vi "Create simplified GUI element.vi"(8 "error in (no error)":errorcluster, 10 "Index":i32, 11 "Optimiser SBlock in":refnum<class "Optimiser SBlock.lvclass">) -> (0 "error out":errorcluster, 2 "Simple GUI Element":T1={"Bcg Color"=16777225, "Index"=0, "No. of runs"=0, "Script name"="", "FPGA name"="", "Parameters"="", "Repetitions"=0}, 3 "Optimiser SBlock out":refnum<class "Optimiser SBlock.lvclass">)   [LabVIEW 2020, in "Run Utilities.lvlib" / "Optimiser SBlock.lvclass"]
doc: "Create a GUI element for this SBlock"
uses:
  Optimiser SBlock.lvclass
  Schedule Block/Schedule Block.lvclass
  Optimiser SBlock.lvclass/Optimiser SBlock.ctl
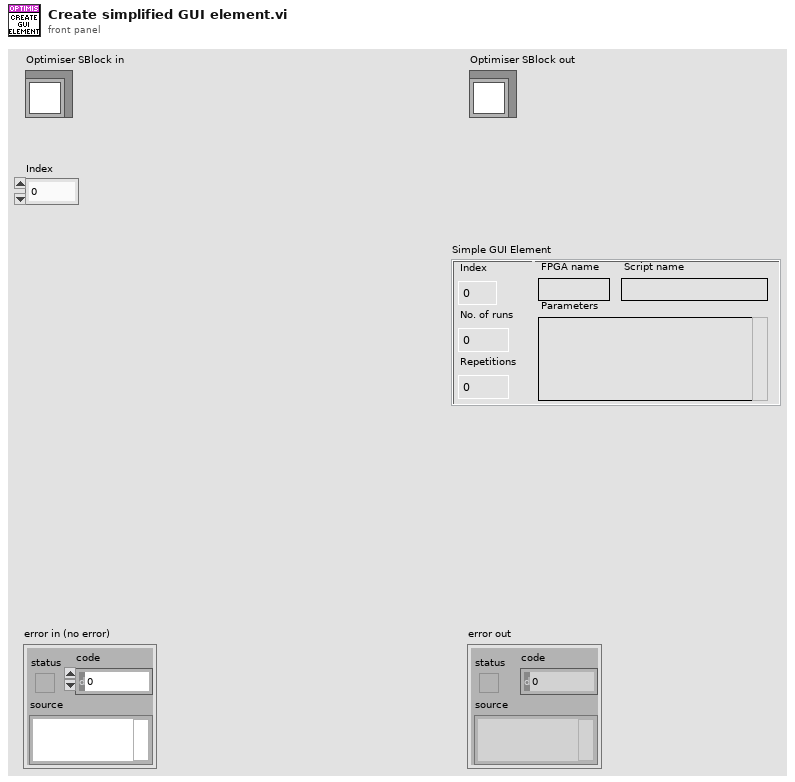
[diagram p1: front panel]
types:
  T1 = cluster{"Bcg Color":u32, "Index":i32, "No. of runs":i32, "Script name":string, "FPGA name":string, "Parameters":string, "Repetitions":i32}
  T2 = typedef "Run Utilities.lvlib/Schedule Block.lvclass/Schedule Block - simplified GUI.ctl" = cluster{"Bcg Color":u32, "Index":i32, "No. of runs":i32, "Script name":string, "FPGA name":string, "Parameters":string, "Repetitions":i32}
  T3 = typedef "Run Utilities.lvlib/Optimiser Cell.lvclass/Optimisation Strategy.ctl" = enum16{"Maximize", "Minimize", "Value"}
  T4 = typedef "Run Utilities.lvlib/Optimiser Cell.lvclass/Optimise parameter - numeric.ctl" = cluster{"Name":string, "Start value":dbl, "From":dbl, "To":dbl, "dtype":enum16{"INT", "DBL"}}
  T5 = typedef "Run Utilities.lvlib/Optimiser Cell.lvclass/Optimise parameter - string.ctl" = cluster{"Name":string, "Start value":string, "Options":string[]}
  T6 = typedef "Run Utilities.lvlib/Optimiser Cell.lvclass/Optimisation observable.ctl" = cluster{"Name":string, "Weight":dbl}
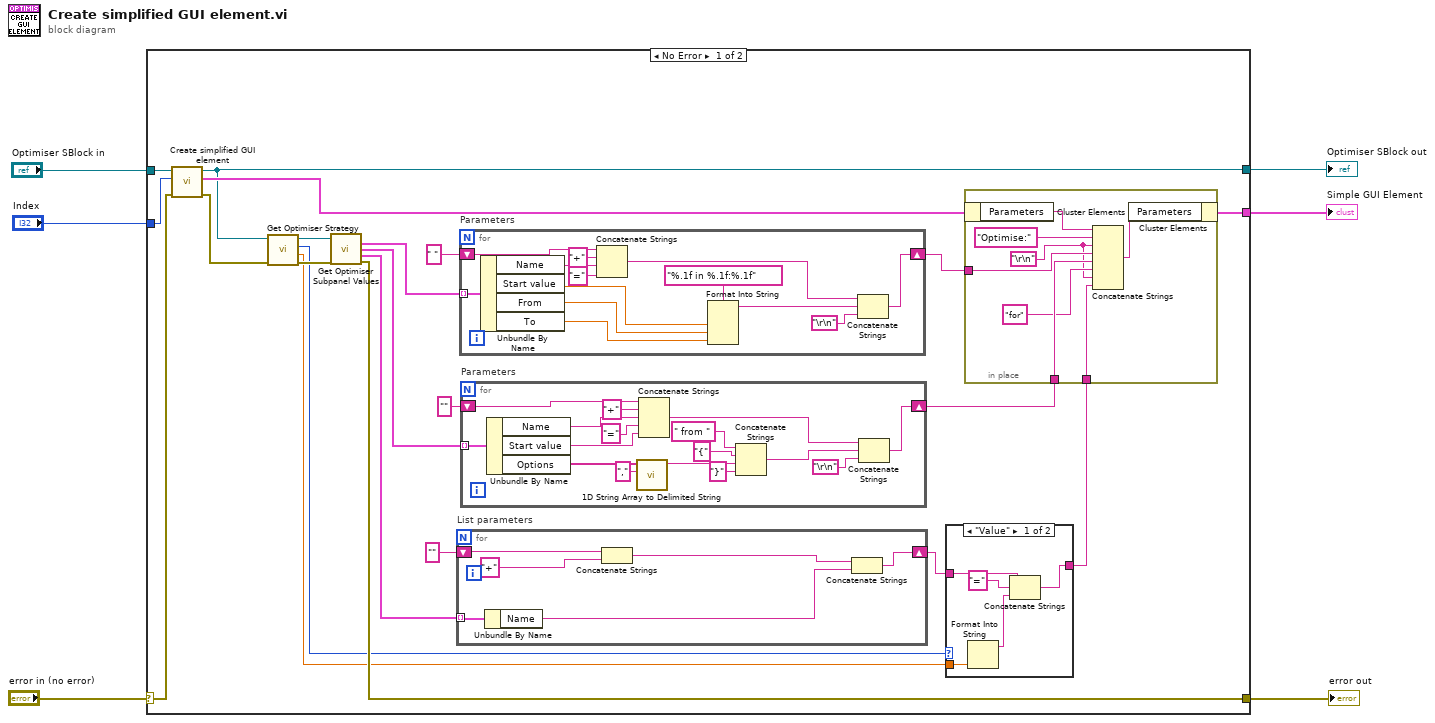
[diagram p0: block diagram]
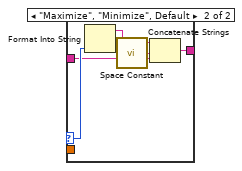
[diagram p2: hidden frame]
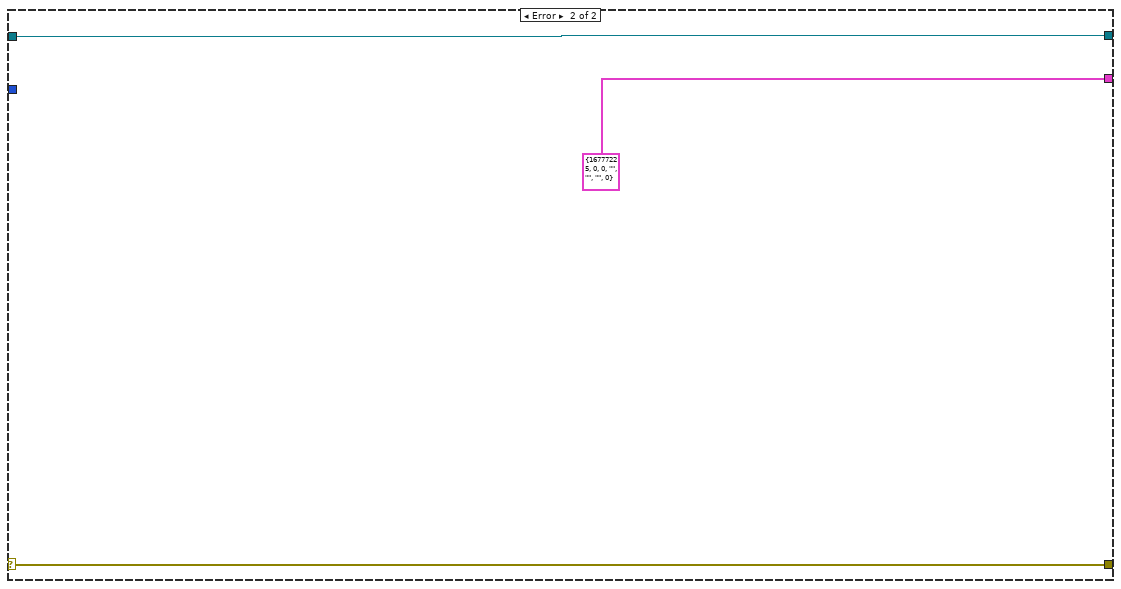
[diagram p3: hidden frame]
diagram:
  n1 = case shown="No Error" "error in (no error)" {
    selector: "error in (no error)" -> [w23 w84]
    tunnel: [w20 w84] -> w1
    tunnel: [w14 w83] -> w3
    tunnel: "Optimiser SBlock in" -> [w25 w83]
    tunnel: [w21 T1 {"Bcg Color"=16777225, "Index"=0, "No. of runs"=0, "Script name"="", "FPGA name"="", "Parameters"="", "Repetitions"=0} ("Cluster")] -> w2
    tunnel: "Index" -> [w24 _]
    frame No Error {
      n2 = call-parent "Create simplified GUI element.vi"("error in (no error)"=w23, "Index"=w24, "Schedule Block in"=w25) -> ("error out"=w13:errorcluster, "Simple GUI Element"=w22:T2, "Schedule Block out"=w14:refnum<class "Optimiser SBlock.lvclass">)  [unwired: 6 in]
      n3 = call-dynamic "Get Optimiser Strategy.vi"("error in (no error)"=w13, "Optimiser SBlock in"=w14) -> ("error out"=w11:errorcluster, "Value"=w7:dbl, "Optimisation Strategy"=w10:T3, "Optimiser SBlock out"=w12:refnum<class "Optimiser SBlock.lvclass">)  [unwired: 6 in]
      n4 = call "Get Optimiser Subpanel Values.vi"("Optimiser SBlock in"=w12, "error in (no error)"=w11) -> ("Parameters - Numeric"=w19:T4[], "Parameters - String"=w16:T5[], "Observables"=w18:T6[], "error out"=w20:errorcluster)  [unwired: 8 in, 2 out]
      n5 = for "List parameters" {
        tunnel: w18 -> [w68] mode=indexing
        shift-right: [w66] -> w9
        shift-left: "" -> [w65]
        n6 = Unbundle By Name(w68) -> ("Name"=w63:string)
        n7 = Concatenate Strings(w65, "+" ("string")) -> (w67:string)
        n8 = Concatenate Strings(w67, w63) -> (w66:string)
      }
      n9 = for "Parameters" {
        tunnel: w19 -> [w81] mode=indexing
        shift-right: [w76] -> w27
        shift-left: " " -> [w75]
        n10 = Unbundle By Name(w81) -> ("Name"=w80:string, "Start value"=w71:dbl, "From"=w69:dbl, "To"=w70:dbl)
        n11 = Concatenate Strings(w75, "+" ("string"), w80, "=" ("string")) -> (w78:string)
        n12 = Format Into String(format string="%.1f in %.1f:%.1f", w71, w69, w70) -> (resulting string=w77:string)  [unwired: 2 in, 1 out]
        n13 = Concatenate Strings(w78, w77, "\r\n") -> (w76:string)
      }
      n14 = for "Parameters" {
        tunnel: w16 -> [w54] mode=indexing
        shift-right: [w50] -> w15
        shift-left: "" -> [w49]
        n15 = Unbundle By Name(w54) -> ("Name"=w53:string, "Start value"=w46:string, "Options"=w45:string[])
        n16 = call <vilib>:"1D String Array to Delimited String.vi"("delimiter"=",", "string array"=w45) -> ("delimited string"=w43:string)  [unwired: 9 in]
        n17 = Concatenate Strings(w49, "+" ("string"), w53, "=" ("string"), w46) -> (w51:string)
        n18 = Concatenate Strings(" from " ("string"), "{" ("string"), w43, "}" ("string")) -> (w40:string)
        n19 = Concatenate Strings(w51, w40, "\r\n") -> (w50:string)
      }
      n20 = case shown="\"Value\"" w10 {
        selector: w10 -> [_ w38]
        tunnel: w9 -> [w33 w36]
        tunnel: [w31 w34] -> w8
        tunnel: w7 -> [w30 _]
        frame "Value" {
          n21 = Format Into String(w30) -> (resulting string=w29:string)  [unwired: 3 in, 1 out]
          n22 = Concatenate Strings(w33, "=" ("string"), w29) -> (w31:string)
        }
        frame "Maximize", "Minimize", Default {
          n23 = Format Into String(w38) -> (resulting string=w37:string)  [unwired: 3 in, 1 out]
          n24 = call <vilib>:"Space Constant.vi"() -> ("String"=w35:string)
          n25 = Concatenate Strings(w37, w35, w36) -> (w34:string)
        }
      }
      n26 = in-place {
        in-place-border: w27 -> [w59]
        in-place-border: w15 -> [w58]
        in-place-border: w8 -> [w55]
        w56 = "\r\n"
        n27 = in-place-cluster #1(w22) -> ("Parameters"=w61:string)
        n28 = Concatenate Strings(w61, "Optimise:" ("string"), w56, w59, w58, "for" ("string"), w56, w55) -> (w60:string)
        n29 = in-place-cluster #1("Parameters"=w60) -> (w21:T2)
      }
    }
    frame Error {
    }
  }
  "error out" <- w1
  "Optimiser SBlock out" <- w3
  "Simple GUI Element" <- w2
